vi "Get Runs.Text.vi"(8 "error in (no error)":errorcluster, 11 "xwpfParagraph in":refnum<class "xwpfParagraph.lvclass">) -> (0 "error out":errorcluster, 2 "Runs.Text":string, 3 "xwpfParagraph out":refnum<class "xwpfParagraph.lvclass">)   [LabVIEW 2017, in "Word_Specific.lvlib" / "xwpfParagraph.lvclass"]
uses:
  xwpfParagraph.lvclass
  xwpfParagraph.lvclass/xwpfParagraph.ctl
  xwpfRun/xwpfRun.lvclass/xwpfRun.ctl
  xwpfRun/Get Text.vi
  xwpfRun/xwpfRun.lvclass
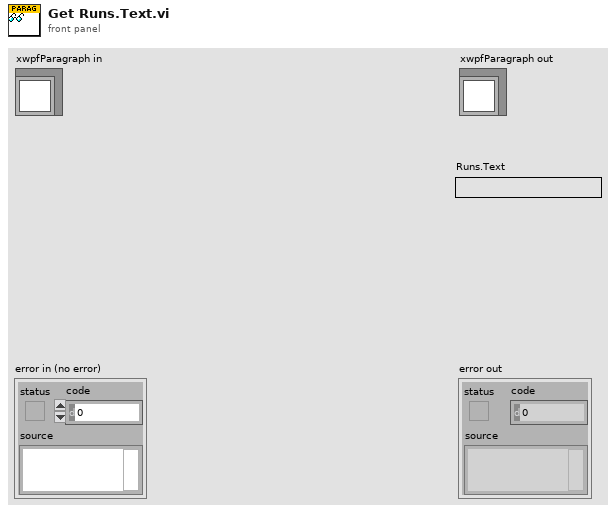
[diagram p1: front panel]
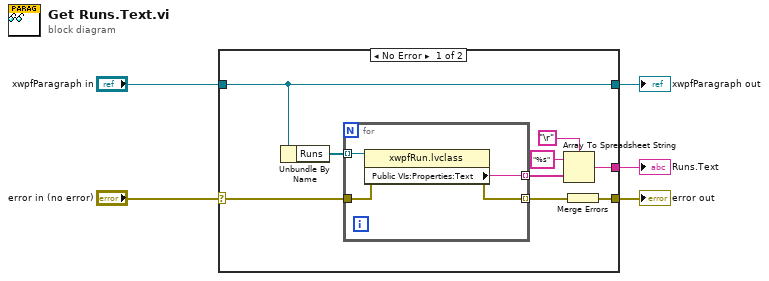
[diagram p0: block diagram]
diagram:
  n1 = case shown="No Error" "error in (no error)" {
    selector: "error in (no error)" -> [w10 w19]
    tunnel: [w11 w19] -> w4
    tunnel: [w14 w20] -> w2
    tunnel: "xwpfParagraph in" -> [w14 w20]
    tunnel: [w8 _] -> w1
    frame No Error {
      n2 = Unbundle By Name(w14) -> ("Runs"=w13:refnum<class "xwpfRun.lvclass">[])
      n3 = for {
        tunnel: w13 -> [w18] mode=indexing
        tunnel: [w17] -> w9 mode=indexing
        tunnel: [w16] -> w12 mode=indexing
        tunnel: w10 -> [w15]
        n4 = property class="xwpfRun.lvclass"(reference=w18, error in=w15) -> (error out=w16:errorcluster, "Public VIs:Properties:Text"=w17:string)  [unwired: 1 out]
      }
      n5 = Array To Spreadsheet String(delimiter (Tab)="\r", array=w9, 3:"%s" ("format string")) -> (spreadsheet string=w8:string)
      n6 = Merge Errors(w12) -> (w11:errorcluster)
    }
    frame Error {
    }
  }
  "error out" <- w4
  "xwpfParagraph out" <- w2
  "Runs.Text" <- w1
